vi "FA_ReadItemXML.vi"(6 "Error In":errorcluster, 8 "Special Type":T1) -> (0 "Error Out":errorcluster, 2 "XML String":string)   [LabVIEW 2014, in "FA_LocalStore.lvlib"]
doc: "Returns the Item XML from LocalStore for a given Special Type."
uses:
  FA_LocalStore.lvlib
  FA_LSSpecialTypes.ctl
  FA_LSCollections.ctl
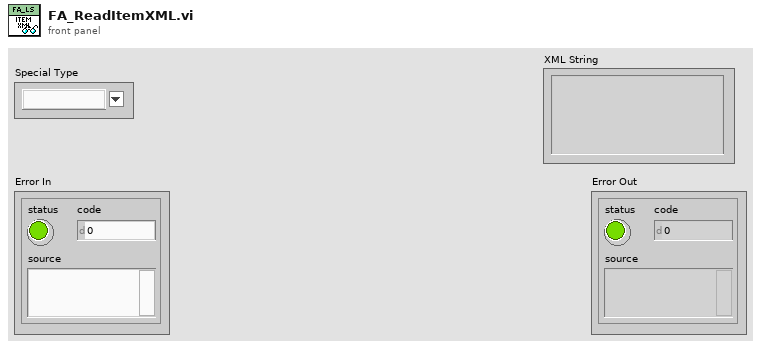
[diagram p1: front panel]
types:
  T1 = typedef "FA_LocalStore.lvlib/FA_LSSpecialTypes.ctl" = string
  T2 = typedef "FA_LocalStore.lvlib/FA_LSCollections.ctl" = enum16{"Config", "ConfigItem", "FA_eTag", "FA_PlugIn"}
  T3 = typedef "FA_LocalStore.lvlib/FA_LSRef.ctl" = cluster{"eTag INI Refnum":T4, "XML Refnum Array":refnum<file>[]}
  T4 = typedef "NI_LVConfig.lvlib/Config Data RefNum.ctl" = refnum<k1>
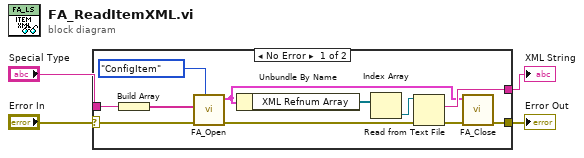
[diagram p0: block diagram]
diagram:
  n1 = case shown="No Error" "Error In" {
    selector: "Error In" -> [w12 w16]
    tunnel: [w7 w16] -> w4
    tunnel: "Special Type" -> [w11 _]
    tunnel: [w15 _] -> w2
    frame No Error {
      n2 = Build Array(w11) -> (w10:T1[])
      n3 = call "FA_Open.vi"("LSCollections"=FA_LSCollections."ConfigItem", "Error In"=w12, "Special Types Array"=w10) -> ("Error Out"=w6:errorcluster, "FA_LS Ref"=w9:T3)  [unwired: 7 in]
      n4 = Unbundle By Name(w9) -> ("XML Refnum Array"=w14:refnum<file>[])
      n5 = Index Array(array=w14) -> (element=w13:refnum<file>)  [unwired: 1 in]
      n6 = Read from Text File(file (use dialog)=w13, error in=w6) -> (text=w15:string, error out=w8:errorcluster)  [unwired: 2 in, 2 out]
      n7 = call "FA_Close.vi"("Error In"=w8, "FA_LS Ref"=w9) -> ("Error Out"=w7:errorcluster)  [unwired: 9 in]
    }
    frame Error {
    }
  }
  "Error Out" <- w4
  "XML String" <- w2
